vi "get update file.vi"(11 "服务器信息":T1={"host"="27.154.58.30", "port"=8020, "user"="std", "password"="std23506", "远端地址"="/微站/室外总磷总氮高压过滤无主板新电路板/一体化微型水质监测站.exe"}) -> ()   [LabVIEW 2016, in "update.lvlib"]
uses:
  update.lvlib
  <vilib>/Utility/error.llb/DialogType.ctl
  <vilib>/httpClient/POSTBuffer.vi
  <vilib>/httpClient/LabVIEWHTTPClient.lvlib
panel:
  out "error out":errorcluster caption="错误输出"
  out "连接的字符串":string
  out "文件大小":i64
  out "headers":string caption="头部"
  out "滑动杆":dbl(slide) scale=0.0..100.0
  out "大小":i64
  out "command":string caption="命令"
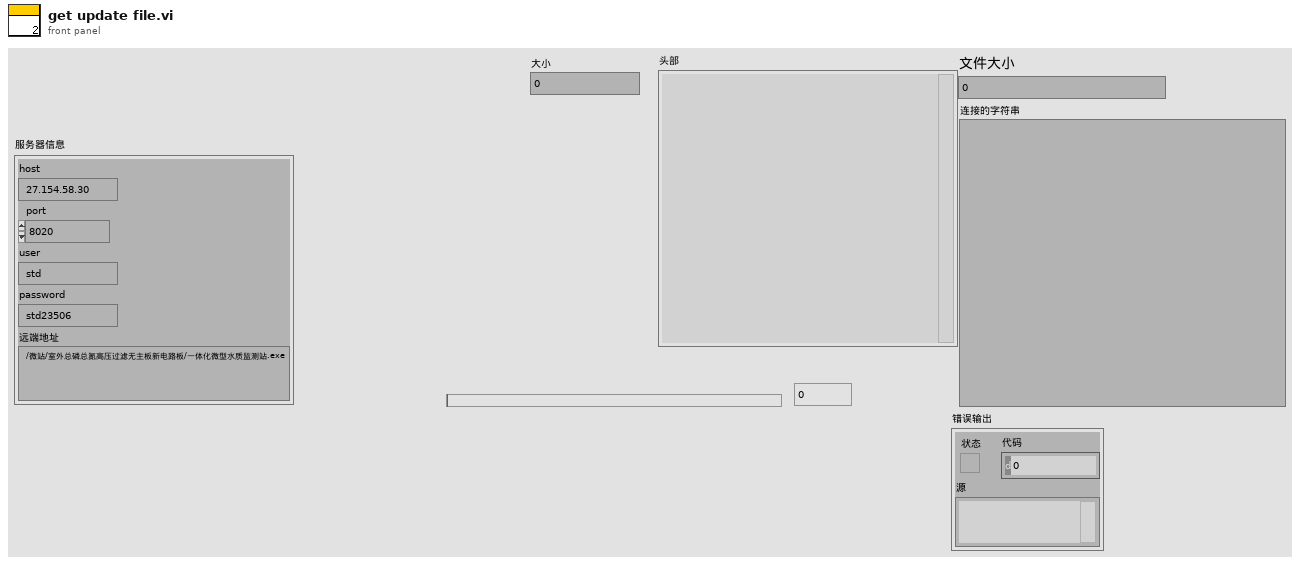
[diagram p1: front panel]
types:
  T1 = cluster{"host":string, "port":u16, "user":string, "password":string, "远端地址":string}
  T2 = enum16{"open", "replace", "create", "open or create", "replace or create", "replace or create with confirmation"}
  T3 = typedef "LabVIEWHTTPClient.lvlib/ClientHandle.ctl" = refnum<k1>
  T4 = typedef "DialogType.ctl" = u16
  T5 = enum32{"invalid app kind", "Development System", "Run Time System", "Student Edition", "Embedded LabVIEW", "Evaluation", "Custom"}
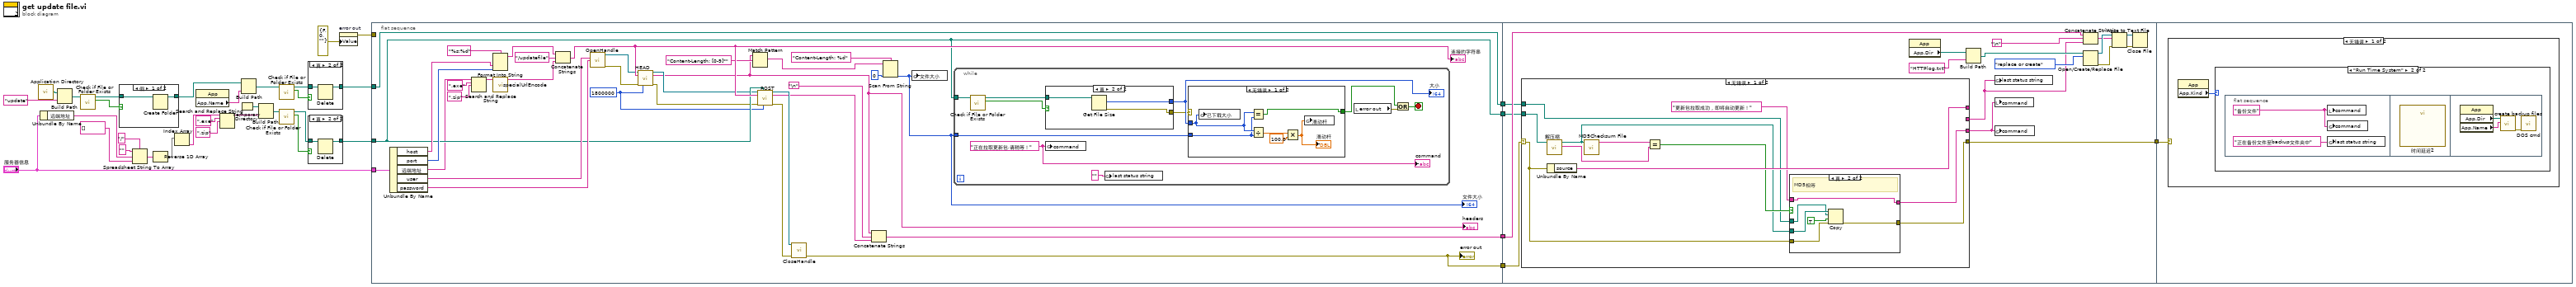
[diagram p0: block diagram]
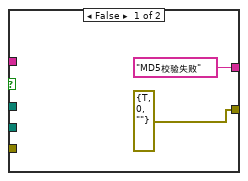
[diagram p7: hidden frame]
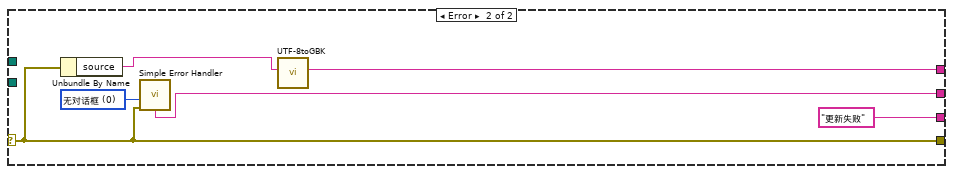
[diagram p8: hidden frame]
diagram:
  n1 = call <vilib>:"Application Directory.vi"() -> ("Application Directory"=w31:path)
  n2 = Unbundle By Name("服务器信息") -> ("远端地址"=w5:string)
  n3 = Build Path(base path=w31, name or relative path="update" ("名称或相对路径")) -> (appended path=w32:path)
  n4 = call <vilib>:"Check if File or Folder Exists.vi"("path"=w32) -> ("file or folder exists?"=w33:bool, "dup path"=w34:path)  [unwired: 8 in, 1 out]
  n5 = case shown="假" w33 {
    tunnel: w34 -> [w36 w37]
    tunnel: [w35 w37] -> w29
    frame False {
      n6 = Create Folder(path (use dialog)=w36) -> (created path=w35:path)  [unwired: 2 in, 2 out]
    }
    frame True {
    }
  }
  n7 = Spreadsheet String To Array(delimiter (Tab)="/" ("分隔符(Tab)"), format string="" ("格式字符串"), spreadsheet string=w5, array type (2D Dbl)=string[] []) -> (array=w3:string[])
  n8 = Reverse 1D Array(array=w3) -> (reversed array=w2:string[])
  n9 = Index Array(array=w2) -> (element=w1:string)  [unwired: 1 in]
  n10 = property class="App"() -> ("App.Name"=w20:string)  [unwired: 2 in, 2 out]
  n11 = Search and Replace String(input string=w1, search string=".exe" ("搜索字符串"), replace string=".zip" ("替换字符串(\"\")")) -> (result string=w24:string)  [unwired: 5 in, 3 out]
  n12 = Temporary Directory() -> (w21:path)
  n13 = Build Path(base path=w29, name or relative path=w20) -> (appended path=w28:path)
  n14 = Build Path(base path=w21, name or relative path=w24) -> (appended path=w10:path)
  n15 = call <vilib>:"Check if File or Folder Exists.vi"("path"=w28) -> ("file or folder exists?"=w27:bool, "dup path"=w26:path)  [unwired: 8 in, 1 out]
  n16 = call <vilib>:"Check if File or Folder Exists.vi"("path"=w10) -> ("file or folder exists?"=w12:bool, "dup path"=w11:path)  [unwired: 8 in, 1 out]
  n17 = case shown="真" w27 {
    tunnel: w26 -> [w38 w40]
    tunnel: [w38 w39] -> w25
    frame False {
    }
    frame True {
      n18 = Delete(path (use dialog)=w40) -> (deleted path=w39:path)  [unwired: 4 in, 2 out]
    }
  }
  n19 = case shown="真" w12 {
    tunnel: w11 -> [w41 w43]
    tunnel: [w41 w42] -> w9
    frame False {
    }
    frame True {
      n20 = Delete(path (use dialog)=w43) -> (deleted path=w42:path)  [unwired: 4 in, 2 out]
    }
  }
  n21 = property on="error out" class="Clust (严格)"("Value"=errorcluster {"status"=FALSE, "code"=0, "source"=""} ("error out")) -> (error out=w14:errorcluster)  [unwired: 2 in, 1 out]
  n22 = flat-sequence {
    tunnel: [w66] -> w19
    tunnel: w25 -> [w63]
    tunnel: "服务器信息" -> [w70]
    tunnel: [w65] -> w18
    tunnel: [w64] -> w17
    tunnel: [w63] -> w16
    tunnel: w9 -> [w64]
    tunnel: w14 -> [_]
    tunnel: w19 -> [w113]
    tunnel: [w99] -> w15
    tunnel: w18 -> [w103]
    tunnel: w17 -> [w98]
    tunnel: w16 -> [w97]
    tunnel: w15 -> [w139]
    frame #0 {
      w49 = 1800000 ("timeout (10000)")
      n23 = Unbundle By Name(w70) -> ("host"=w74:string, "port"=w73:u16, "远端地址"=w60:string, "user"=w69:string, "password"=w68:string)
      n24 = Search and Replace String(input string=w60, search string=".exe" ("搜索字符串"), replace string=".zip" ("替换字符串(\"\")")) -> (result string=w59:string)  [unwired: 5 in, 3 out]
      n25 = Format Into String(format string="%s:%d" ("格式字符串"), w74, w73) -> (resulting string=w72:string)  [unwired: 2 in, 1 out]
      n26 = call "specialUrlEncode.vi"("str"=w59) -> ("UrlEncode"=w75:string)  [unwired: 10 in]
      n27 = Concatenate Strings(w72, "/updatefile", w75) -> (w67:string)
      "连接的字符串" <- w67
      n28 = call <vilib>:"OpenHandle.vi"("username"=w69, "password"=w68) -> ("client handle out"=w53:T3, "error out"=w51:errorcluster)  [unwired: 12 in]
      n29 = call <vilib>:"HEAD.vi"("client handle"=w53, "url"=w67, "error in (no error)"=w51, "timeout (10000)"=w49) -> ("client handle out"=w52:T3, "headers"=w44:string, "error out"=w50:errorcluster)  [unwired: 9 in]
      "headers" <- w44
      n30 = Match Pattern(string=w44, regular expression="Content-Length: [0-9]*") -> (match substring=w47:string)  [unwired: 1 in, 3 out]
      n31 = call-poly <vilib>:"POST.vi"("client handle"=w52, "output file"=w64, "url"=w67, "error in (no error)"=w50, "timeout (10000)"=w49) -> ("client handle out"=w56:T3, "headers"=w54:string, "error out"=w55:errorcluster)  [unwired: 7 in, 1 out]
      n32 = call <vilib>:"CloseHandle.vi"("client handle"=w56, "error in (no error)"=w55) -> ("error out"=w66:errorcluster)  [unwired: 13 in]
      "error out" <- w66
      n33 = Concatenate Strings(w44, "\n", w54) -> (w65:string)
      n34 = Scan From String(format string="Content-Length: %d", input string=w47, default 1=i64 0 ("default value 1")) -> (output 1=w58:i64)  [unwired: 2 in, 3 out]
      "文件大小" <- w58
      n35 = global write "更新全局变量.vi" "文件大小"(w58) -> ()
      n36 = while {
        tunnel: w64 -> [w79]
        tunnel: w58 -> [w84]
        stop <- w82 stop-if-true
        w86 = "正在拉取更新包,请稍等！" ("格式字符串")
        n37 = call <vilib>:"Check if File or Folder Exists.vi"("path"=w79) -> ("file or folder exists?"=w77:bool, "dup path"=w78:path)  [unwired: 8 in, 1 out]
        n38 = case shown="真" w77 {
          tunnel: [_ w90] -> w87
          tunnel: [_ w89] -> w83
          tunnel: w78 -> [_ w88]
          frame False {
          }
          frame True {
            n39 = Get File Size(file=w88) -> (size (in bytes)=w90:i64, 0:w89:errorcluster)  [unwired: 1 in, 1 out]
          }
        }
        "大小" <- w87
        n40 = global write "更新全局变量.vi" "command"(w86) -> ()
        n41 = global write "更新全局变量.vi" "last status string"("" ("last status string")) -> ()
        n42 = case shown="无错误" w83 {
          tunnel: w87 -> [w93 _]
          tunnel: w84 -> [w92 _]
          tunnel: [w91 _] -> w81
          frame No Error {
            n43 = global write "更新全局变量.vi" "已下载大小"(w93) -> ()
            n44 = Equal?(x=w93, y=w92) -> (x = y?=w91:bool)
            n45 = Divide(x=w93, y=w92) -> (x/y=w96:dbl)
            n46 = Multiply(x=w96, y=100.0) -> (x*y=w95:dbl)
            "滑动杆" <- w95
            n47 = global write "更新全局变量.vi" "滑动杆"(w95) -> ()
          }
          frame Error {
          }
        }
        n48 = local read "error out"() -> (w80:errorcluster)
        n49 = Compound Arithmetic op=OR ("复合运算")(w81, w80) -> (w82:bool)
        "command" <- w86
      }
    }
    frame #1 {
      n50 = case shown="无错误" w113 {
        selector: w113 -> [w118 w133]
        tunnel: [w120 "更新失败" ("command")] -> w112
        tunnel: [w124 w136] -> _
        tunnel: [_ w134] -> w100
        tunnel: [w119 w133] -> w99
        tunnel: w98 -> [w117 _]
        tunnel: w97 -> [w114 _]
        frame No Error {
          n51 = call "解压缩.vi"("Zip file"=w117) -> ("MD5"=w116:string, "待校验的文件路径"=w115:path)  [unwired: 8 in, 1 out]
          n52 = Unbundle By Name(w118) -> ("source"=w124:string)
          n53 = call <vilib>:"MD5Checksum File.vi"("Path"=w115) -> ("MD5 message-digest"=w123:string)  [unwired: 9 in, 1 out]
          n54 = Equal?(x=w123, y=w116) -> (x = y?=w122:bool)
          n55 = case shown="真" w122 {
            tunnel: ["MD5校验失败" w132] -> w120
            tunnel: "更新包拉取成功，即将自动更新！" ("command") -> [_ w132]
            tunnel: [errorcluster {"status"=TRUE, "code"=0, "source"=""} ("error IO") w129] -> w119
            tunnel: w118 -> [_ w130]
            tunnel: w115 -> [_ w128]
            tunnel: w114 -> [_ w127]
            frame False {
            }
            frame True {
              # "MD5相等"
              n56 = Copy(8:w130, 9:TRUE ("覆盖(F)"), 10:w127, 11:w128) -> (0:w129:errorcluster)  [unwired: 1 in, 2 out]
            }
          }
        }
        frame Error {
          w135 = T4 0 items=["无对话框", "确定信息", "继续或停止信息", "确定信息＋警告", "继续/停止+警告"] ("type of dialog (OK msg:1)")
          n57 = Unbundle By Name(w133) -> ("source"=w137:string)
          n58 = call <vilib>:"Simple Error Handler.vi"("type of dialog (OK msg:1)"=w135, "error in (no error)"=w133) -> ("message"=w134:string)  [unwired: 3 in, 4 out]
          n59 = call "UTF-8toGBK.vi"("UTF-8"=w137) -> ("GBK"=w136:string)  [unwired: 9 in, 1 out]
        }
      }
      n60 = property class="App"() -> ("App.Dir"=w105:path)  [unwired: 2 in, 2 out]
      n61 = Build Path(base path=w105, name or relative path="HTTPlog.txt" ("名称或相对路径")) -> (appended path=w107:path)
      n62 = global write "更新全局变量.vi" "last status string"(w100) -> ()
      n63 = local write "command"(w112) -> ()
      n64 = global write "更新全局变量.vi" "command"(w112) -> ()
      n65 = Concatenate Strings(w103, "\n", w100) -> (w101:string)
      n66 = Open/Create/Replace File(file path (use dialog)=w107, operation (0:open)=T2."replace or create" ("操作(0:open)")) -> (refnum out=w110:refnum<file>, error out=w109:errorcluster)  [unwired: 4 in, 1 out]
      n67 = Write to Text File(file (use dialog)=w110, text=w101, error in=w109) -> (refnum out=w111:refnum<file>, error out=w104:errorcluster)  [unwired: 1 in, 1 out]
      n68 = Close File(refnum=w111, error in=w104) -> ()  [unwired: 2 out]
    }
    frame #2 {
      n69 = case shown="无错误" w139 {
        frame No Error {
          n70 = property class="App"() -> ("App.Kind"=w140:T5)  [unwired: 2 in, 2 out]
          n71 = case shown="\"Run Time System\"" w140 {
            frame "invalid app kind", Default {
            }
            frame "Run Time System" {
              n72 = flat-sequence {
                frame #0 {
                  w142 = "备份文件" ("command")
                  n73 = local write "command"(w142) -> ()
                  n74 = global write "更新全局变量.vi" "command"(w142) -> ()
                  n75 = global write "更新全局变量.vi" "last status string"("正在备份文件至backup文件夹中" ("last status string")) -> ()
                }
                frame #1 {
                  n76 = call "时间延迟2"() -> ()  [unwired: 11 in, 1 out]
                }
                frame #2 {
                  n77 = property class="App"() -> ("App.Dir"=w145:path, "App.Name"=w144:string)  [unwired: 2 in, 2 out]
                  n78 = call "create backup files.vi"("execute file name"=w144, "路径"=w145) -> ("error out"=w143:errorcluster)  [unwired: 9 in]
                  n79 = call "DOS cmd.vi"("错误输入（无错误）"=w143) -> ()  [unwired: 10 in, 1 out]
                }
              }
            }
          }
        }
        frame Error {
        }
      }
    }
  }
